vi "send_standard_to_AnalysisObj.vi"(0 "SessionID":string, 5 "standard_name":string, 7 "standard_type":string, 9 "Isotope Table":cluster{"isotope":string, "amount cc":dbl}[](array[cluster]), 11 "error in (no error)":errorcluster) -> (15 "error out":errorcluster)   [LabVIEW 2017]
doc: "sendds the data to the AnalysisSession (SessionID) and stores them in the AnalysisDataArray"
uses:
  global variables.vi
  Classes/StatusLog/StatusLog.lvclass
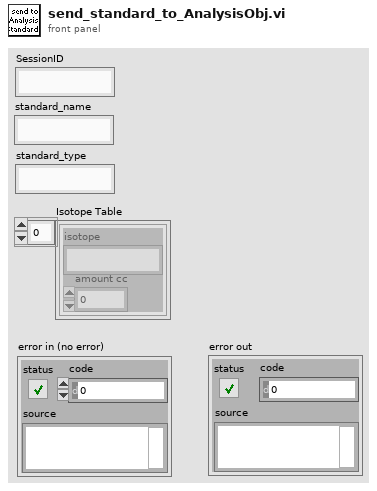
[diagram p1: front panel]
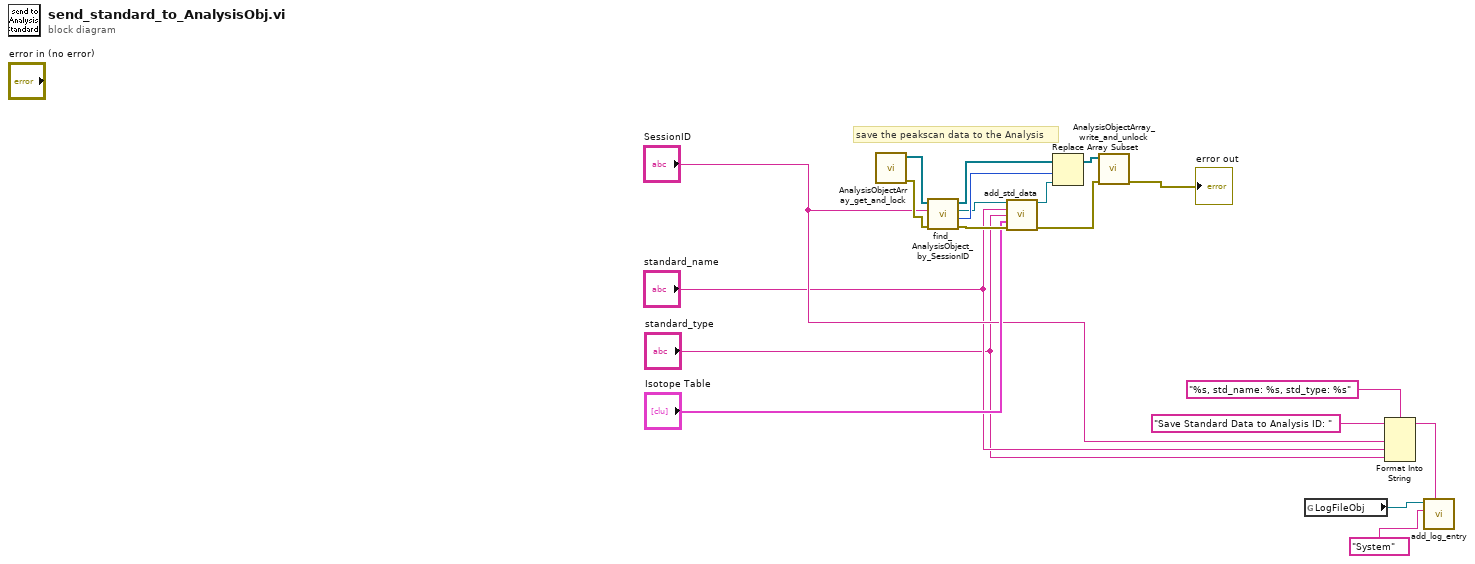
[diagram p0: block diagram]
diagram:
  # "save the peakscan data to the Analysis"
  n1 = call "AnalysisObjectArray_get_and_lock.vi"() -> ("error out"=w15:errorcluster, "AnalysisObjects"=w14:refnum<class "Analysis.lvclass">[])  [unwired: 10 in]
  n2 = call "find_AnalysisObject_by_SessionID.vi"("error in (no error)"=w15, "SessionID"="SessionID", "AnalysisObjects in"=w14) -> ("error out"=w13:errorcluster, "index of found"=w17:i32, "found AnalyisObject"=w10:refnum<class "Analysis.lvclass">, "AnalysisObjects out"=w16:refnum<class "Analysis.lvclass">[])  [unwired: 5 in]
  n3 = call "add_std_data.vi"("Analysis in"=w10, "standard_name"="standard_name", "standard_type"="standard_type", "Isotope Table"="Isotope Table", "error in (no error)"=w13) -> ("Analysis out"=w12:refnum<class "Analysis.lvclass">, "error out"=w11:errorcluster)  [unwired: 9 in]
  n4 = Replace Array Subset(array=w16, new element=w12, index=w17) -> (w18:refnum<class "Analysis.lvclass">[])
  n5 = call "AnalysisObjectArray_write_and_unlock.vi"("error in (no error)"=w11, "AnalysisObjects"=w18) -> ("error out"=→"error out":errorcluster)  [unwired: 9 in]
  n6 = global read "global variables.vi" "LogFileObj"() -> (w9:refnum<class "StatusLog.lvclass">)
  n7 = Format Into String(format string="%s, std_name: %s, std_type: %s", initial string="Save Standard Data to Analysis ID: ", "SessionID", "standard_name", "standard_type") -> (resulting string=w1:string)  [unwired: 1 in, 1 out]
  n8 = call-dynamic "add_log_entry.vi"("new entry"=w1, "log identifiers"="System", "StatusLog in"=w9) -> ()  [unwired: 5 in, 2 out]
